vi "demarcate_qupingjun.vi"() -> ()   [LabVIEW 2020]
uses:
  <vilib>/Analysis/baseanly.llb/Mean (DBL).vi
  <vilib>/Utility/file.llb/Read Delimited Spreadsheet (DBL).vi
  <vilib>/Analysis/NI_AALBase.lvlib
panel:
  out "平均":dbl
  out "大小":i32[](array[numeric])
  in  "file path (dialog if empty)":path caption="文件路径 （空时为对话框）"
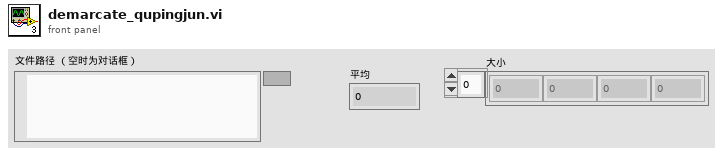
[diagram p1: front panel]
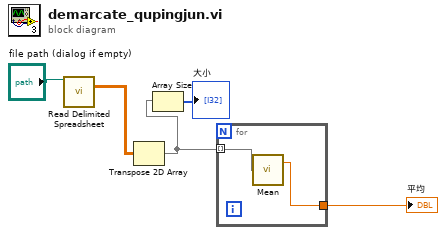
[diagram p0: block diagram]
diagram:
  n1 = call-poly <vilib>:"Read Delimited Spreadsheet.vi"("file path (dialog if empty)"="file path (dialog if empty)") -> ("all rows"=w2:dbl[][])  [unwired: 9 in, 5 out]
  n2 = Transpose 2D Array(2D array=w2) -> (transposed array=w1:dbl[][])
  n3 = Array Size(array=w1) -> (size(s)=→"大小":i32[])
  n4 = for {
    tunnel: [w7] -> w3
    tunnel: w1 -> [w6] mode=indexing
    n5 = call-poly <vilib>:"Mean.vi"("X"=w6) -> ("mean"=w7:dbl)  [unwired: 1 out]
  }
  "平均" <- w3
